vi "GetHelp.vi"(11 "LUnitCLI In":refnum<class "LUnitCLI.lvclass">) -> (2 "Help":string, 3 "LUnitCLI Out":refnum<class "LUnitCLI.lvclass">)   [LabVIEW 2020, in "LUnitCLI.lvclass"]
uses:
  LUnitCLI.lvclass
  LUnitCLI.lvclass/LUnitCLI.ctl
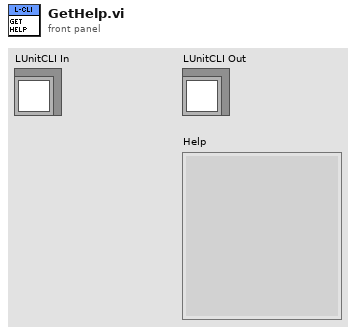
[diagram p1: front panel]
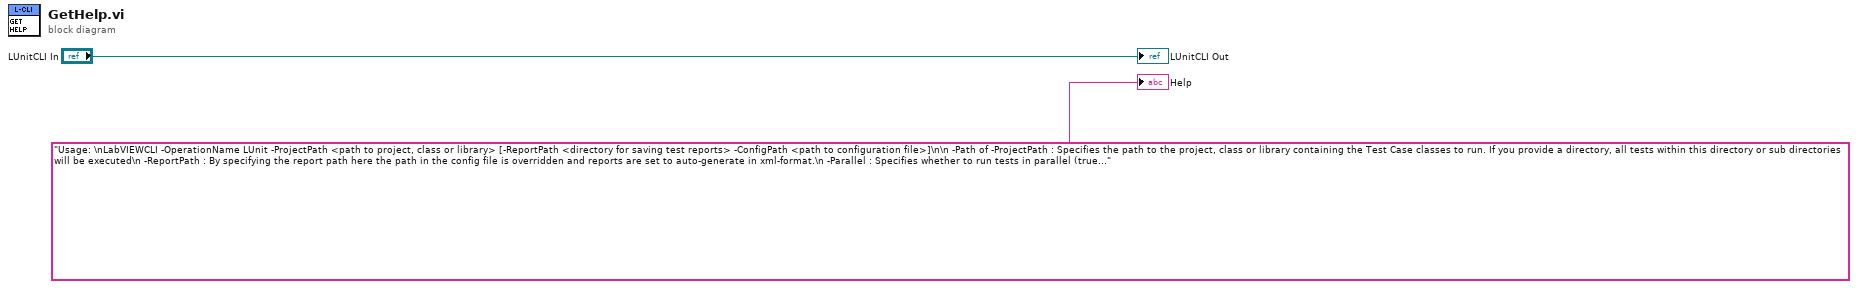
[diagram p0: block diagram]
diagram:
  "LUnitCLI Out" <- "LUnitCLI In"
  "Help" <- "Usage: \nLabVIEWCLI -OperationName LUnit -ProjectPath <path to project, class or library> [-ReportPath <directory for saving test reports> -ConfigPath <path to configuration file>]\n\n -Path of -ProjectPath : Specifies the path to the project, class or library containing the Test Case classes to run. If you provide a directory, all tests within this directory or sub directories will be executed\n -ReportPath : By specifying the report path here the path in the config file is overridden and reports are set to auto-generate in xml-format.\n -Parallel : Specifies whether to run tests in parallel (true or false). Default is false.\n -TestRunners : Specifies the number of parallell test runners to spawn. Default value is 1. This is an alias for Parallel. Any value >1 will have same result as \"-Prallel true\"\n -ClearIndex : Clear the index and force LUnit to rediscover all tests. Default is True.\n -CustomReports: If there are custom report plugins installed, these can be activated by providing them as a comma separated list. If this is left empty, the default plugin will be selected based on the given file extenssion. If any of the built-in reporting formats (Text Report or XML Report) should stil be active, they should be added to the list. "
